vi "浊度_所有参数读取.vi"(8 "error in (no error)":errorcluster caption="错误输入（无错误）", 11 "MB session in":refnum<class "MB_Master.lvclass">) -> (0 "error out":errorcluster caption="错误输出", 2 "输出值":T1 {"电极型号标志" items=["NULL", "pH", "Cond", "DO", "Turb"]; "电极状态标志" items=["OK"=0, "第一点校正通过"=1, "第二点校正通过"=2, "悬浮物两点校准第一点校正通过"=11, "悬浮物两点校准第二点校正通过"=12, "浊度三点校正第一点校正通过"=31, "浊度三点校正第二点校正通过"=32, "浊度三点校正第三点校正通过"=33]}, 3 "MB session out":refnum<class "MB_Master.lvclass">)   [LabVIEW 2016, in "斯坦道多参数.lvlib"]
uses:
  <vilib>/Plasmionique/MB Master/MB_Master/MB_Master.lvclass
  <vilib>/Plasmionique/MB Master/MB Master.lvlib
  <vilib>/ptbypt/NI_PtbyPt.lvlib
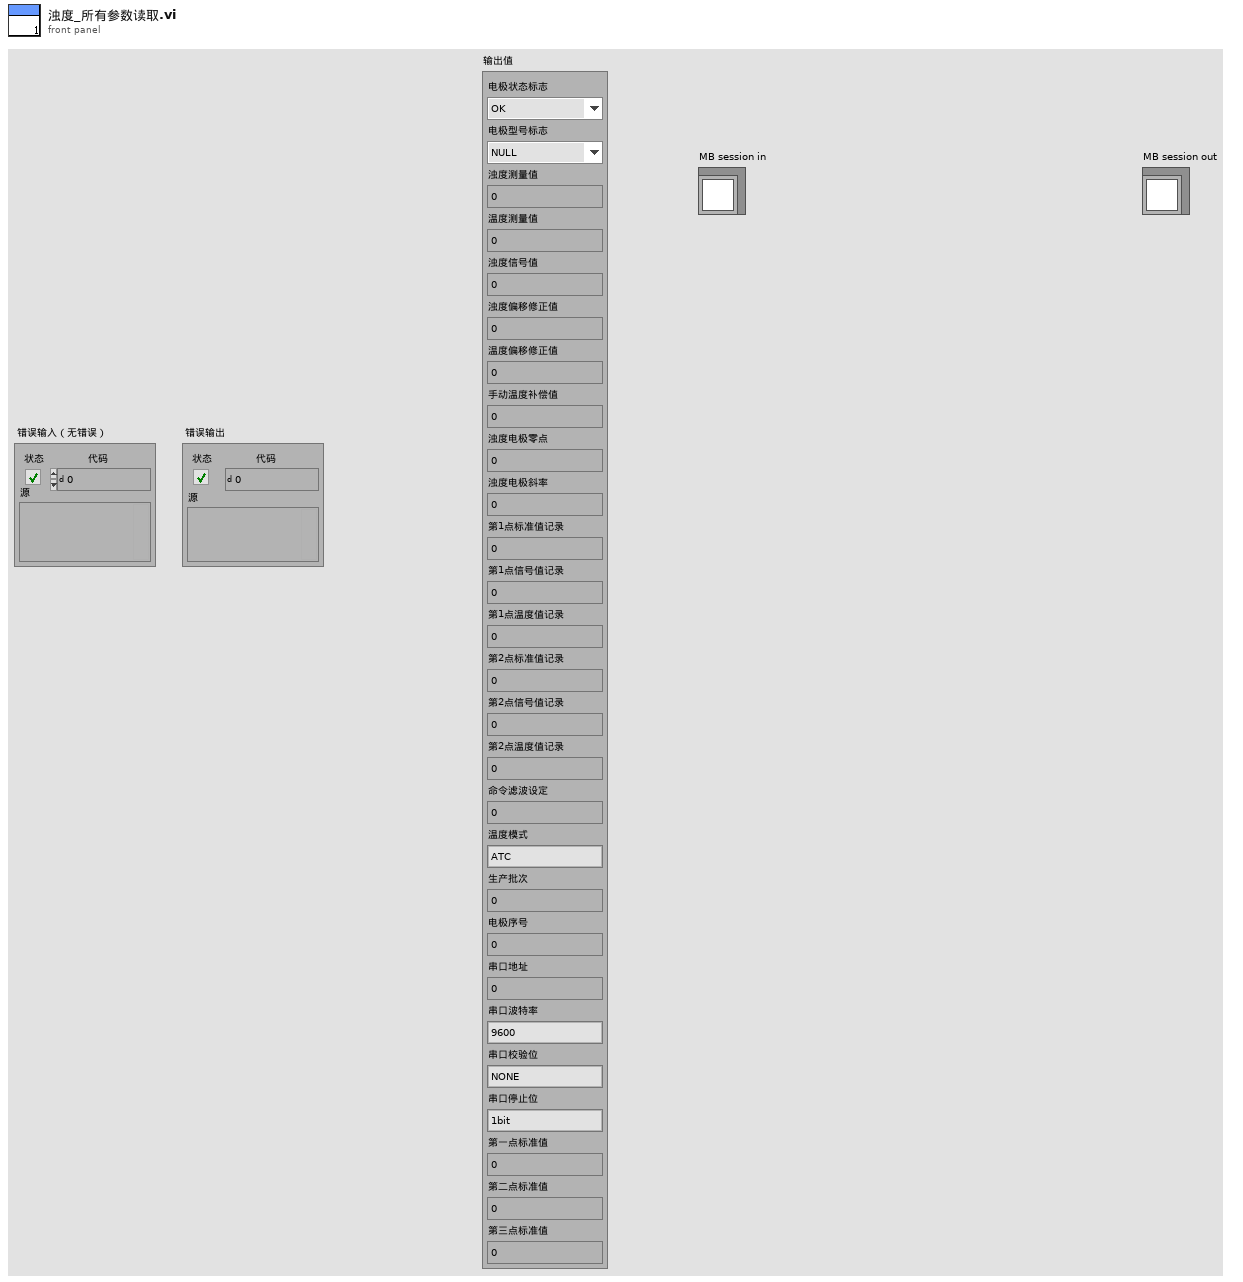
[diagram p1: front panel]
types:
  T1 = cluster{"电极状态标志":u16, "电极型号标志":u16, "浊度测量值":sgl, "温度测量值":sgl, "浊度信号值":sgl, "浊度偏移修正值":sgl, "温度偏移修正值":sgl, "手动温度补偿值":sgl, "浊度电极零点":sgl, "浊度电极斜率":sgl, "第1点标准值记录":sgl, "第1点信号值记录":sgl, "第1点温度值记录":sgl, "第2点标准值记录":sgl, "第2点信号值记录":sgl, "第2点温度值记录":sgl, "命令滤波设定":u16, "温度模式":enum16{"ATC", "MTC"}, "生产批次":u16, "电极序号":u16, "串口地址":u16, "串口波特率":enum16{"9600", "19200", "115200"}, "串口校验位":enum16{"NONE", "ODD", "EVEN"}, "串口停止位":enum16{"1bit", "2bit"}, "第一点标准值":sgl, "第二点标准值":sgl, "第三点标准值":sgl}
  T2 = cluster{u16, u16, "Filtered x":dbl, "数值":sgl, "数值":sgl, "数值":sgl, "数值":sgl, "数值":sgl, "数值":sgl, "数值":sgl, "数值":sgl, "数值":sgl, "数值":sgl, "数值":sgl, "数值":sgl, "数值":sgl, u16, u16, u16, u16, u16, u16, u16, u16, "数值":sgl, "数值":sgl, "数值":sgl}
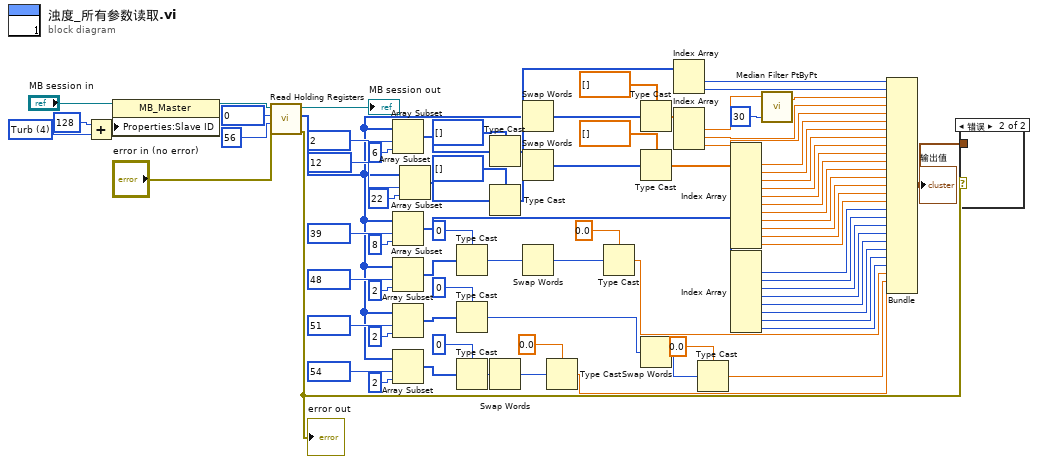
[diagram p0: block diagram]
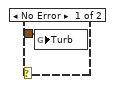
[diagram p2: hidden frame]
diagram:
  w81 = u16 4 items=["NULL", "pH", "Cond", "DO", "Turb"] ("数值")
  n1 = Add(x=u16 128, y=w81) -> (x+y=w80:u16)
  n2 = property class="MB_Master"(reference="MB session in", "Properties:Slave ID"=w80) -> (reference out=w17:refnum<class "MB_Master.lvclass">)  [unwired: 1 in, 1 out]
  n3 = call <vilib>:"Read Holding Registers.vi"("error in (no error)"="error in (no error)", "quantity"=u16 56, "starting address"=u16 0, "MB session in"=w17) -> ("error out"=w16:errorcluster, "Registers"=w7:u16[], "MB session out"=→"MB session out":refnum<class "MB_Master.lvclass">)  [unwired: 5 in]
  "error out" <- w16
  n4 = Array Subset(array=w7, index=u16 2 ("starting address"), length=6 ("长度")) -> (w69:u16[])
  n5 = Array Subset(array=w7, index=u16 39 ("starting address"), length=8 ("长度")) -> (w43:u16[])
  n6 = Array Subset(array=w7, index=u16 48 ("starting address"), length=2 ("长度")) -> (w26:u16[])
  n7 = Array Subset(array=w7, index=u16 51 ("starting address"), length=2 ("长度")) -> (w21:u16[])
  n8 = Array Subset(array=w7, index=u16 54 ("starting address"), length=2 ("长度")) -> (w14:u16[])
  n9 = Array Subset(array=w7, index=u16 12 ("starting address"), length=22 ("长度")) -> (w60:u16[])
  n10 = Type Cast(type=u32 0 ("数值"), x=w26) -> (*(type *) &x=w29:u32)
  n11 = Type Cast(type=u32 0 ("数值"), x=w21) -> (*(type *) &x=w23:u32)
  n12 = Type Cast(type=u32 0 ("数值"), x=w14) -> (*(type *) &x=w12:u32)
  n13 = Type Cast(type=u32[] [] ("数组 2"), x=w69) -> (*(type *) &x=w71:u32[])
  n14 = Type Cast(type=u32[] [] ("数组 2"), x=w60) -> (*(type *) &x=w63:u32[])
  n15 = Swap Words(1:w12) -> (0:w13:u32)
  n16 = Swap Words(1:w71) -> (0:w73:u32[])
  n17 = Swap Words(1:w63) -> (0:w64:u32[])
  n18 = Swap Words(1:w29) -> (0:w30:u32)
  n19 = Type Cast(type=sgl 0.0 ("数值"), x=w13) -> (*(type *) &x=w6:sgl)
  n20 = Type Cast(type=sgl 0.0 ("数值"), x=w30) -> (*(type *) &x=w20:sgl)
  n21 = Type Cast(type=sgl[] [] ("数组 2"), x=w73) -> (*(type *) &x=w68:sgl[])
  n22 = Type Cast(type=sgl[] [] ("数组 2"), x=w64) -> (*(type *) &x=w59:sgl[])
  n23 = Swap Words(1:w23) -> (0:w22:u32)
  n24 = Index Array(array=w7) -> (element #1=w76:u16, element #2=w75:u16)  [unwired: 2 in]
  n25 = Index Array(array=w68) -> (element #1=w2:sgl, element #2=w67:sgl, element #3=w66:sgl)  [unwired: 3 in]
  n26 = Type Cast(type=sgl 0.0 ("数值"), x=w22) -> (*(type *) &x=w19:sgl)
  n27 = Index Array(array=w59) -> (element #1=w58:sgl, element #2=w57:sgl, element #3=w56:sgl, element #4=w55:sgl, element #5=w54:sgl, element #6=w53:sgl, element #7=w52:sgl, element #8=w51:sgl, element #9=w50:sgl, element #10=w49:sgl, element #11=w48:sgl)  [unwired: 11 in]
  n28 = Index Array(array=w43) -> (element #1=w42:u16, element #2=w41:u16, element #3=w40:u16, element #4=w39:u16, element #5=w38:u16, element #6=w37:u16, element #7=w36:u16, element #8=w35:u16)  [unwired: 8 in]
  n29 = call <vilib>:"Median Filter PtByPt.vi"("rank"=30, "x"=w2) -> ("Filtered x"=w1:dbl)  [unwired: 2 in, 1 out]
  n30 = Bundle(w76, w75, "Filtered x"=w1, "数值"=w67, "数值"=w66, "数值"=w58, "数值"=w57, "数值"=w56, "数值"=w55, "数值"=w54, "数值"=w53, "数值"=w52, "数值"=w51, "数值"=w50, "数值"=w49, "数值"=w48, w42, w41, w40, w39, w38, w37, w36, w35, "数值"=w20, "数值"=w19, "数值"=w6) -> (w15:T2)  [unwired: 1 in]
  "输出值" <- w15
  n31 = case shown="错误" w16 {
    tunnel: w15 -> [w82 _]
    frame No Error {
      n32 = global write "国弘过程全局变量.vi" "Turb"(w82) -> ()
    }
    frame Error {
    }
  }
